vi "Wait for Callback.vi"(8 "error in (no error)":errorcluster, 9 "timeout in ms (-1)":i32=-1, 11 "Synchronous Request Callback In":refnum<class "Synchronous Request Callback.lvclass">) -> (0 "error out":errorcluster, 1 "timed out?":bool, 2 "notification":T1, 3 "Synchronous Request Callback Out":refnum<class "Synchronous Request Callback.lvclass">)   [LabVIEW 2020, in "Synchronous Request Callback.lvclass"]
uses:
  Synchronous Request Callback.lvclass
  Synchronous Request Callback.lvclass/Synchronous Request Callback.ctl
  Process/Protected/Messaging/Response Message Cluster.ctl
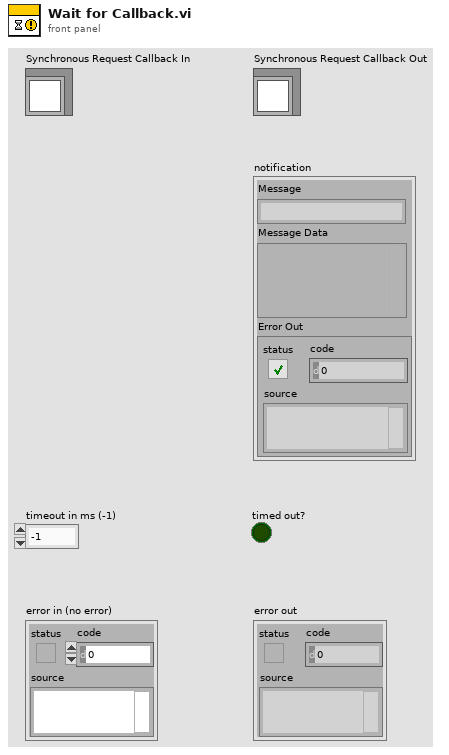
[diagram p1: front panel]
types:
  T1 = typedef "Synchronous Request Callback.lvclass/Response Message Cluster.ctl" = cluster{"Message":string, "Message Data":variant, "Error Out":errorcluster}
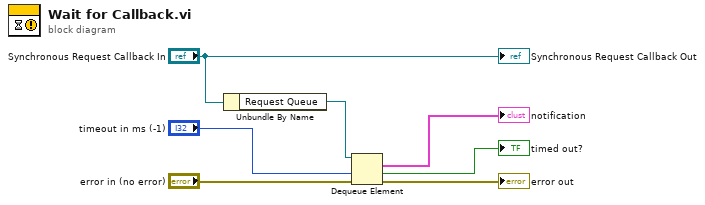
[diagram p0: block diagram]
diagram:
  n1 = Unbundle By Name("Synchronous Request Callback In") -> ("Request Queue"=w4:refnum<queue>)
  n2 = Dequeue Element(queue=w4, timeout in ms (-1)="timeout in ms (-1)", error in (no error)="error in (no error)") -> (element=→"notification":T1, timed out?=→"timed out?":bool, error out=→"error out":errorcluster)  [unwired: 1 out]
  "Synchronous Request Callback Out" <- "Synchronous Request Callback In"
